vi "Disconnect Relays connected to site.vi"(0 "TSM context":T1, 11 "error in":errorcluster) -> (4 "TSM context out":T1, 15 "error out":errorcluster)   [LabVIEW 2019]
uses:
  <vilib>/NI_TestStand_SemiconductorModule/NI_TestStand_Semiconductor_Module.lvlibp/PinMap/General/SemiconductorModuleContext.ctl
  <vilib>/NI_TestStand_SemiconductorModule/NI_TestStand_Semiconductor_Module.lvlibp/PinMap/Relay Driver/ApplyRelayConfiguration.vi
  <vilib>/NI_TestStand_SemiconductorModule/NI_TestStand_Semiconductor_Module.lvlibp
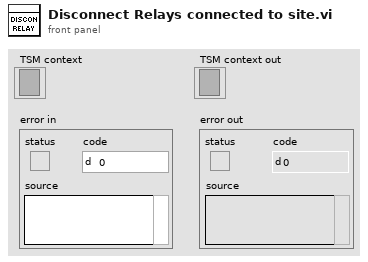
[diagram p1: front panel]
types:
  T1 = typedef "NI_TestStand_Semiconductor_Module.lvlibp/SemiconductorModuleContext.ctl" = refnum<k7>
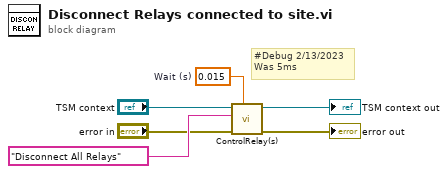
[diagram p0: block diagram]
diagram:
  w1 = 0.015  # Wait (s)
  # "#Debug 2/13/2023\nWas 5ms"
  n1 = call-poly <vilib>:"ControlRelay(s).vi"("Wait (s)"=w1, "error in (no error)"="error in", "Relay Configuration"=tag "Disconnect All Relays", "Semiconductor Module Context"="TSM context") -> ("error out"=→"error out":errorcluster, "Semiconductor Module Context Out"=→"TSM context out":T1)  [unwired: 6 in]
